vi "Python List to Array of Elements.vi"(8 "error in (no error)":errorcluster, 10 "Python List":string) -> (0 "error out":errorcluster, 2 "Elements":string[](array[string]))   [LabVIEW 2020, in "jki_python_data_tools.lvlib"]
uses:
  jki_python_data_tools.lvlib
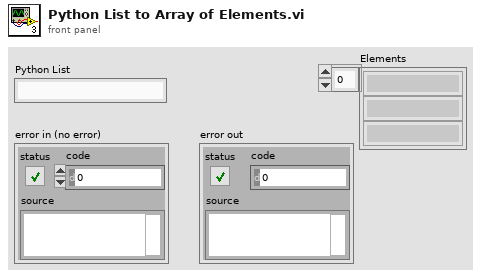
[diagram p1: front panel]
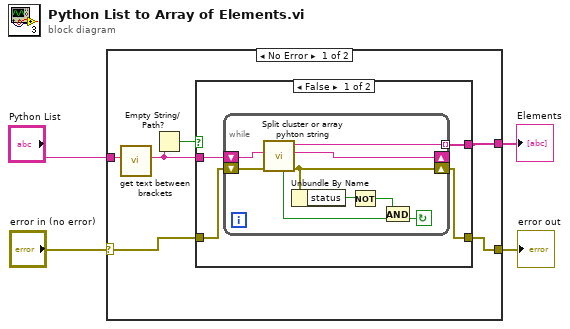
[diagram p0: block diagram]
diagram:
  n1 = case shown="No Error" "error in (no error)" {
    selector: "error in (no error)" -> [w5 w25]
    tunnel: [w10 w25] -> w4
    tunnel: [w9 _] -> w3
    tunnel: "Python List" -> [w8 _]
    frame No Error {
      n2 = call "get text between brackets.vi"("Python String"=w8) -> ("Text Between Brakets"=w6:string)  [unwired: 10 in]
      n3 = Empty String/Path?(string/path=w6) -> (empty?=w7:bool)
      n4 = case shown="False" w7 {
        tunnel: [w14 w24] -> w10
        tunnel: w5 -> [w13 w24]
        tunnel: [w12 _] -> w9
        tunnel: w6 -> [w11 _]
        frame False {
          n5 = while {
            shift-right: [w22] -> _
            shift-left: w11 -> [w21]
            tunnel: [w23] -> w12 mode=indexing
            shift-right: [w18] -> w14
            shift-left: w13 -> [w19]
            stop <- w16 continue-if-true
            n6 = call "Split cluster or array pyhton string.vi"("error in (no error)"=w19, "Comma Delimited Python Data"=w21) -> ("error out"=w18:errorcluster, "Remaining Elements"=w22:string, "First Element"=w23:string, "Has Remaining Elements"=w20:bool)  [unwired: 5 in, 1 out]
            n7 = Unbundle By Name(w18) -> ("status"=w17:bool)
            n8 = Not(x=w17) -> (.not. x?=w15:bool)
            n9 = And(x=w15, y=w20) -> (x .and. y?=w16:bool)
          }
        }
        frame True {
        }
      }
    }
    frame Error {
    }
  }
  "error out" <- w4
  "Elements" <- w3
